vi "Init Lidar.vi"(8 "error in (no error)":errorcluster) -> (0 "error out":errorcluster)   [LabVIEW 2017]
uses:
  MyRIO/VI/Private/Send acquisition command.vi
  MyRIO/VI/Private/Enable Laser.vi
  MyRIO/VI/Private/Open Lidar.vi
  MyRIO/VI/Private/Init shared library.vi
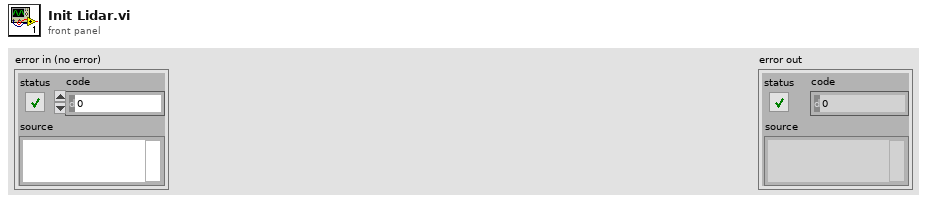
[diagram p1: front panel]
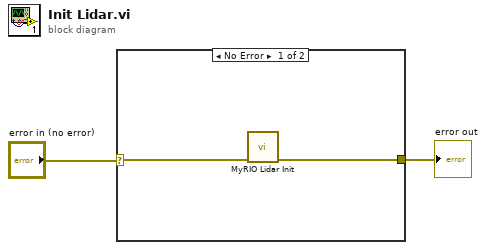
[diagram p0: block diagram]
diagram:
  n1 = case shown="No Error" "error in (no error)" {
    selector: "error in (no error)" -> [w3 w5]
    tunnel: [w4 w5] -> w2
    frame No Error {
      n2 = call "MyRIO Lidar Init.vi"("error in (no error)"=w3) -> ("error out"=w4:errorcluster)  [unwired: 10 in]
    }
    frame Error {
    }
  }
  "error out" <- w2
